vi "NEW数据采集传输系统.vi"() -> ()   [LabVIEW 2016, in "数据传输系统-06.lvlib"]
uses:
  <vilib>/Utility/miscctls.llb/LVPointTypeDef.ctl
  <vilib>/Utility/error.llb/whitespace.ctl
  <vilib>/picture/picture.llb/imagedata.ctl
  <vilib>/Utility/config.llb/NI_LVConfig.lvlib
  update/update.lvlib
panel:
  in  "共享MN":bool
  out "剖面数据补发":bool
  out "日志信息补发":bool
  out "数据补发":bool
  in  "自动更新":bool
  in  "数据补传":bool caption="确定"
  out "数据库打开失败次数":dbl
  out "与工控通信指示灯":bool
  in  "判断数据反馈":enum16{"非严格判断", "严格判断", "不判断"}(ring)
  in  "暂停上传":bool
  in  "配置表":bool caption="确定"
  in  "updateconfiguration":T1={"主机"="27.154.58.30", "用户"="update", "密码"="std23506", "远程路径"="数据传输系统\\平台数据传输系统.exe", "下载文件名"="平台数据传输系统.exe", "软件版本"=""}
  out "标题显示":string
  in  "更新":bool
  in  "系统编码选择框":string(combo)="地表水质量监测"
  in  "数据发送通道":enum16{"TCP", "VISA"}(ring)
  in  "baud rate":u32=9600 caption="波特率"
  in  "VISA resource name":refnum<visa-resource-name> caption="VISA资源名称"
  in  "实时数据发送时间间隔/min":i32=1
  in  "数据组合发送":bool
  in  "2011发送":bool
  in  "数据发送协议":enum16{"2005-212协议", "2017-212协议"}(ring)=enum."2017-212协议"
  in  "重发时间":T2(ring)
  in  "重发日期":T3(ring)
  in  "开机启动":bool
  in  "每周自动重发":bool=TRUE
  in  "确定":bool
  in  "返回":bool
  in  "PW":string
  in  "MN":string
  in  "PORT":string
  in  "IP":string
  in  "站点设备":string
  in  "站点名称":string
  out "设置超时时间/min":i32=1
  out "状态信息":T4={"1st Error to Convert "=63, "步骤 "=enum."发送数据", "元素"="实时数据", "TCP服务端掉线计数"=0, "TCP掉线时间节点"="2019/05/08 15:24:17"} {"1st Error to Convert" items=["无错误", "参数错误", "内存已满", "超出区域", "文件结束", "文件已打开", "一般文件IO错误", "未找到文件", "文件权限错误", "磁盘已满", "路径副本", "打开过多文件", "未启用", "未找到资源文件", "无法添加资源", "未找到资源", "未找到图像", "图像内存错误", "画笔不存在", "配置错误类型", "配置未找到解析段", "配置解析错误", "配置内存错误", "错误外部代码格式", "错误外部代码偏移量", "外部代码不存在", "空窗口", "销毁窗口错误", "空菜单", "打印已中止", "错误打印记录", "打印驱动程序错误", "打印时窗口错误", "打印时内存错误", "打印对话框错误", "一般打印错误", "无效设备引用句柄", "设备未找到", "设备参数错误", "设备单位错误", "无法打开设备", "设备调用已中止", "一般错误", "用户已取消", "对象ID过低", "对象ID过高", "对象不在堆中", "未知的堆", "错误DefProc ID", "DefProc不在表格中", "范围外信息", "空方法", "未知信息", "不支持管理器调用", "错误地址", "连接过程中", "连接超时", "连接过程中", "不支持网络属性", "网络错误", "正在使用的地址", "系统缺少内存", "连接已中止", "连接已拒绝", "连接未建立", "连接已建立", "连接已关闭", "初始化错误（交互应用程序管理器）", "错误事件发生", "等待无约束事件发生处理程序", "事件发生队列溢出", "错误路径", "未发出信号量", "未识别类型（交互应用程序管理器）"]}
  out "数据接收超时指示灯":bool
  out "空闲时间/s":string
  out "系统时间":string
  out "实时小时数据上传":bool
  out "系统状态改变":bool
  out "软件版本":string
  out "掉线指示":bool
  out "核查数据上传":bool
  out "配置信息":T5
  in  "参数配置":bool
  out "反控数据发送":bool
  out "读取报文显示":string
  out "发送报文显示":string
  out "心跳包":bool
  out "通信状态":bool
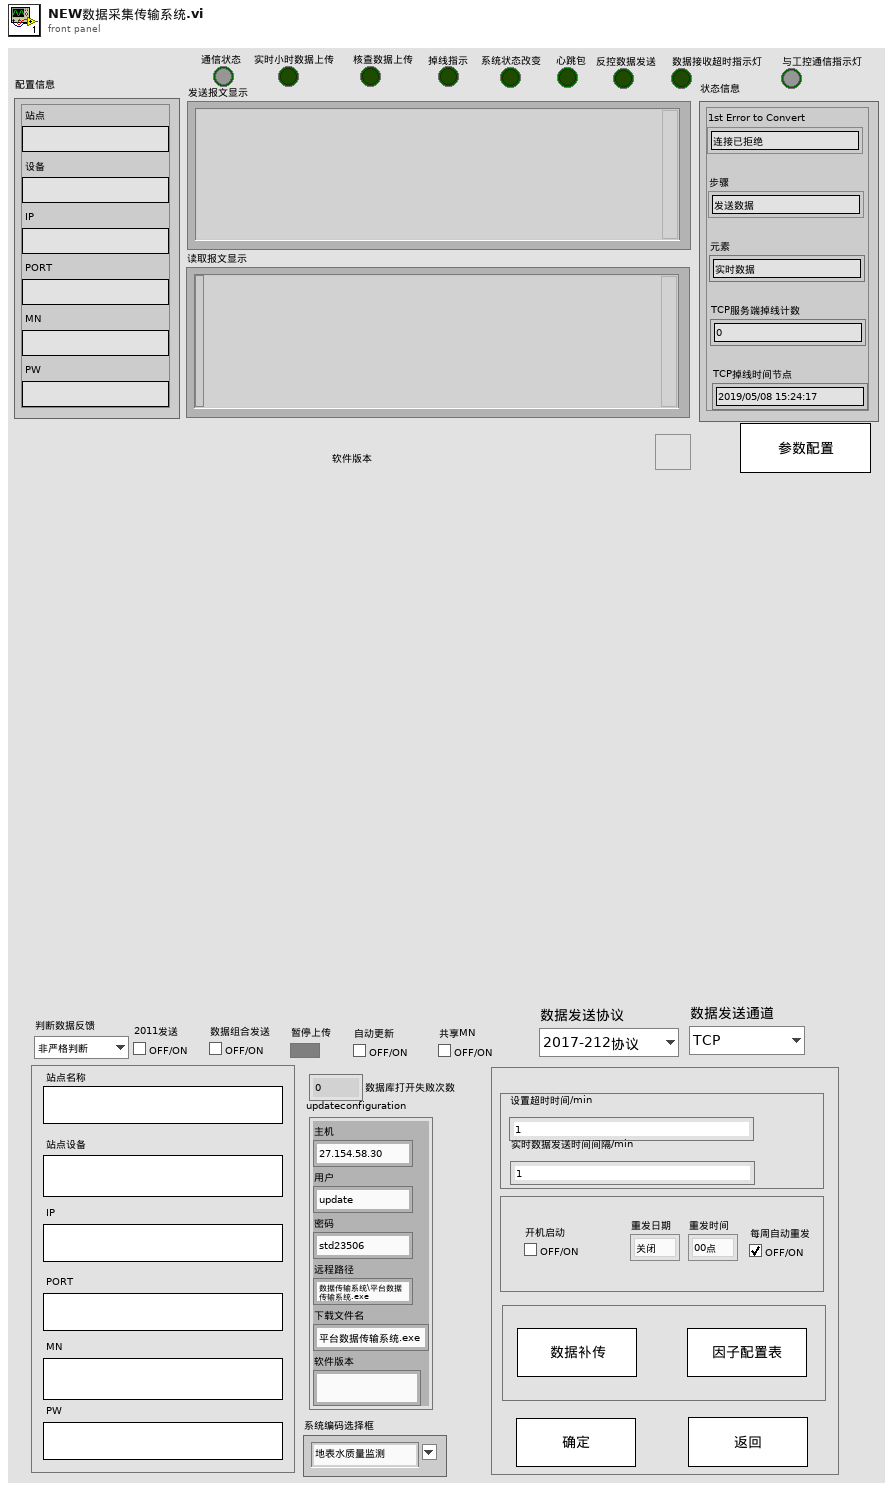
[diagram p1: front panel]
types:
  T1 = cluster{"主机":string, "用户":string, "密码":string, "远程路径":string, "下载文件名":string, "软件版本":string}
  T2 = enum16{"00点", "01点", "02点", "03点", "04点", "05点", "06点", "07点", "08点", "09点", "10点", "11点", "12点", "13点", "14点", "15点", "16点", "17点", "18点", "19点", "20点", "21点", "22点", "23点"}
  T3 = enum16{"关闭", "星期日", "星期一", "星期二", "星期三", "星期四", "星期五", "星期六"}
  T4 = cluster{"1st Error to Convert ":i32, "步骤 ":enum16{"打开连接", "发送数据", "读取数据", "数据处理", "关闭连接"}, "元素":string, "TCP服务端掉线计数":i32, "TCP掉线时间节点":string}
  T5 = cluster{"站点":string, "设备":string, "IP":string, "PORT":string, "MN":string, "PW":string}
  T6 = typedef "imagedata.ctl" = cluster{"image type":i32, "image depth":i32, "image":u8[], "mask":u8[], "colors":u32[], "Rectangle":cluster{"left":i16, "top":i16, "right":i16, "bottom":i16}}
  T7 = typedef "LVPointTypeDef.ctl" = cluster{"Horizontal":i16, "Vertical":i16}
  T8 = cluster{"setini":string, "sysini":string, "hechaini":string, "actualwrite":string, "actualread":string, "datasent":string, "反控命令信息队列":string, "反控与仪器交互":string}
  T9 = cluster{"配置表格[0]":string, "配置表格[1]":string, "配置表格[2]":string, "配置表格[3]":string, "配置表格[4]":string, "配置表格[5]":string, "配置表格[6]":string, "配置表格[7]":string, "配置表格[8]":string, "配置表格[9]":string, "配置表格[10]":string, "配置表格[11]":string, "配置表格[12]":string, "配置表格[13]":string, "配置表格[14]":string, "配置表格[15]":string, "配置表格[16]":string, "配置表格[17]":string, "配置表格[18]":string, "配置表格[19]":string, "配置表格[20]":string, "配置表格[21]":string, "配置表格[22]":string, "配置表格[23]":string, "配置表格[24]":string, "配置表格[25]":string, "配置表格[26]":string, "配置表格[27]":string, "配置表格[28]":string, "配置表格[29]":string, "配置表格[30]":string, "配置表格[31]":string, "配置表格[32]":string, "配置表格[33]":string, "配置表格[34]":string, "配置表格[35]":string, "配置表格[36]":string}
  T10 = cluster{"[0]":dbl, "[1]":dbl, "[2]":dbl, "[3]":dbl, "[4]":dbl, "[5]":dbl, "[6]":dbl, "[7]":dbl, "[8]":dbl, "[9]":dbl, "[10]":dbl, "[11]":dbl, "[12]":dbl, "[13]":dbl, "[14]":dbl, "[15]":dbl, "[16]":dbl, "[17]":dbl, "[18]":dbl, "[19]":dbl, "[20]":dbl, "[21]":dbl, "[22]":dbl, "[23]":dbl, "[24]":dbl, "[25]":dbl, "[26]":dbl, "[27]":dbl, "[28]":dbl, "[29]":dbl, "[30]":dbl, "[31]":dbl, "[32]":dbl, "[33]":dbl, "[34]":dbl, "[35]":dbl, "[36]":dbl}
  T11 = cluster{"时间标识":timestamp, "设备":string, "日志信息":string, "流程参数":string}
  T12 = typedef "NI_LVConfig.lvlib/Config Data RefNum.ctl" = refnum<k1>
  T13 = cluster{"CODMn":bool, "CODCr":bool, "DO":bool, "铜":bool, "PH":bool, "氨氮":bool, "比电导率":bool, "水温":bool, "COD":bool, "浊度":bool, "总氮":bool, "总磷":bool, "叶绿素a":bool, "藻密度":bool, "水位":bool, "流速":bool, "瞬时流量":bool, "累积流量":bool, "亚硝氮":bool, "硫化物":bool, "ORP":bool, "铅":bool, "镉":bool, "锌":bool, "镍":bool, "锰":bool, "汞":bool, "气温":bool, "气压":bool, "风速":bool, "风向":bool, "盐度":bool, "磷酸盐":bool, "硝氮":bool, "氟化物":bool, "挥发酚":bool, "氯化物":bool}
  T14 = cluster{"time1":string, "time2":string, "time3":string, "time4":string, "time5":string, "time6":string, "time7":string, "time8":string, "time9":string, "time10":string, "time11":string, "time12":string, "time13":string, "time14":string, "time15":string, "time16":string, "time17":string, "time18":string, "time19":string, "time20":string, "time21":string, "time22":string, "time23":string, "time24":string, "time25":string, "time26":string, "time27":string, "time28":string, "time29":string, "time30":string, "time31":string, "time32":string, "time33":string, "time34":string, "time35":string, "time36":string, "time37":string}
  T15 = cluster{"[0]":string, "[1]":string, "[2]":string, "[3]":string, "[4]":string, "[5]":string, "[6]":string, "[7]":string}
  T16 = cluster{"[0]":string, "[1]":string, "[2]":string, "[3]":string, "[4]":string, "[5]":string, "[6]":string, "[7]":string, "[8]":string, "[9]":string}
  T17 = cluster{"[0]":string, "[1]":string, "[2]":string, "[3]":string, "[4]":string, "[5]":string, "[6]":string}
  T18 = cluster{"[0]":string, "[1]":string, "[2]":string, "[3]":string, "[4]":string, "[5]":string, "[6]":string, "[7]":string, "[8]":string, "[9]":string, "[10]":string, "[11]":string, "[12]":string, "[13]":string, "[14]":string, "[15]":string, "[16]":string, "[17]":string}
  T19 = cluster{"[0]":string, "[1]":string, "[2]":string, "[3]":string, "[4]":string, "[5]":string, "[6]":string, "[7]":string, "[8]":string, "[9]":string, "[10]":string, "[11]":string, "[12]":string, "[13]":string, "[14]":string}
  T20 = cluster{"[0]":string, "[1]":string, "[2]":string, "[3]":string, "[4]":string, "[5]":string, "[6]":string, "[7]":string, "[8]":string, "[9]":string, "[10]":string, "[11]":string, "[12]":string, "[13]":string, "[14]":string, "[15]":string, "[16]":string, "[17]":string, "[18]":string, "[19]":string, "[20]":string, "[21]":string, "[22]":string, "[23]":string, "[24]":string, "[25]":string, "[26]":string, "[27]":string, "[28]":string, "[29]":string, "[30]":string, "[31]":string, "[32]":string, "[33]":string, "[34]":string, "[35]":string, "[36]":string}
  T21 = typedef "whitespace.ctl" = u16
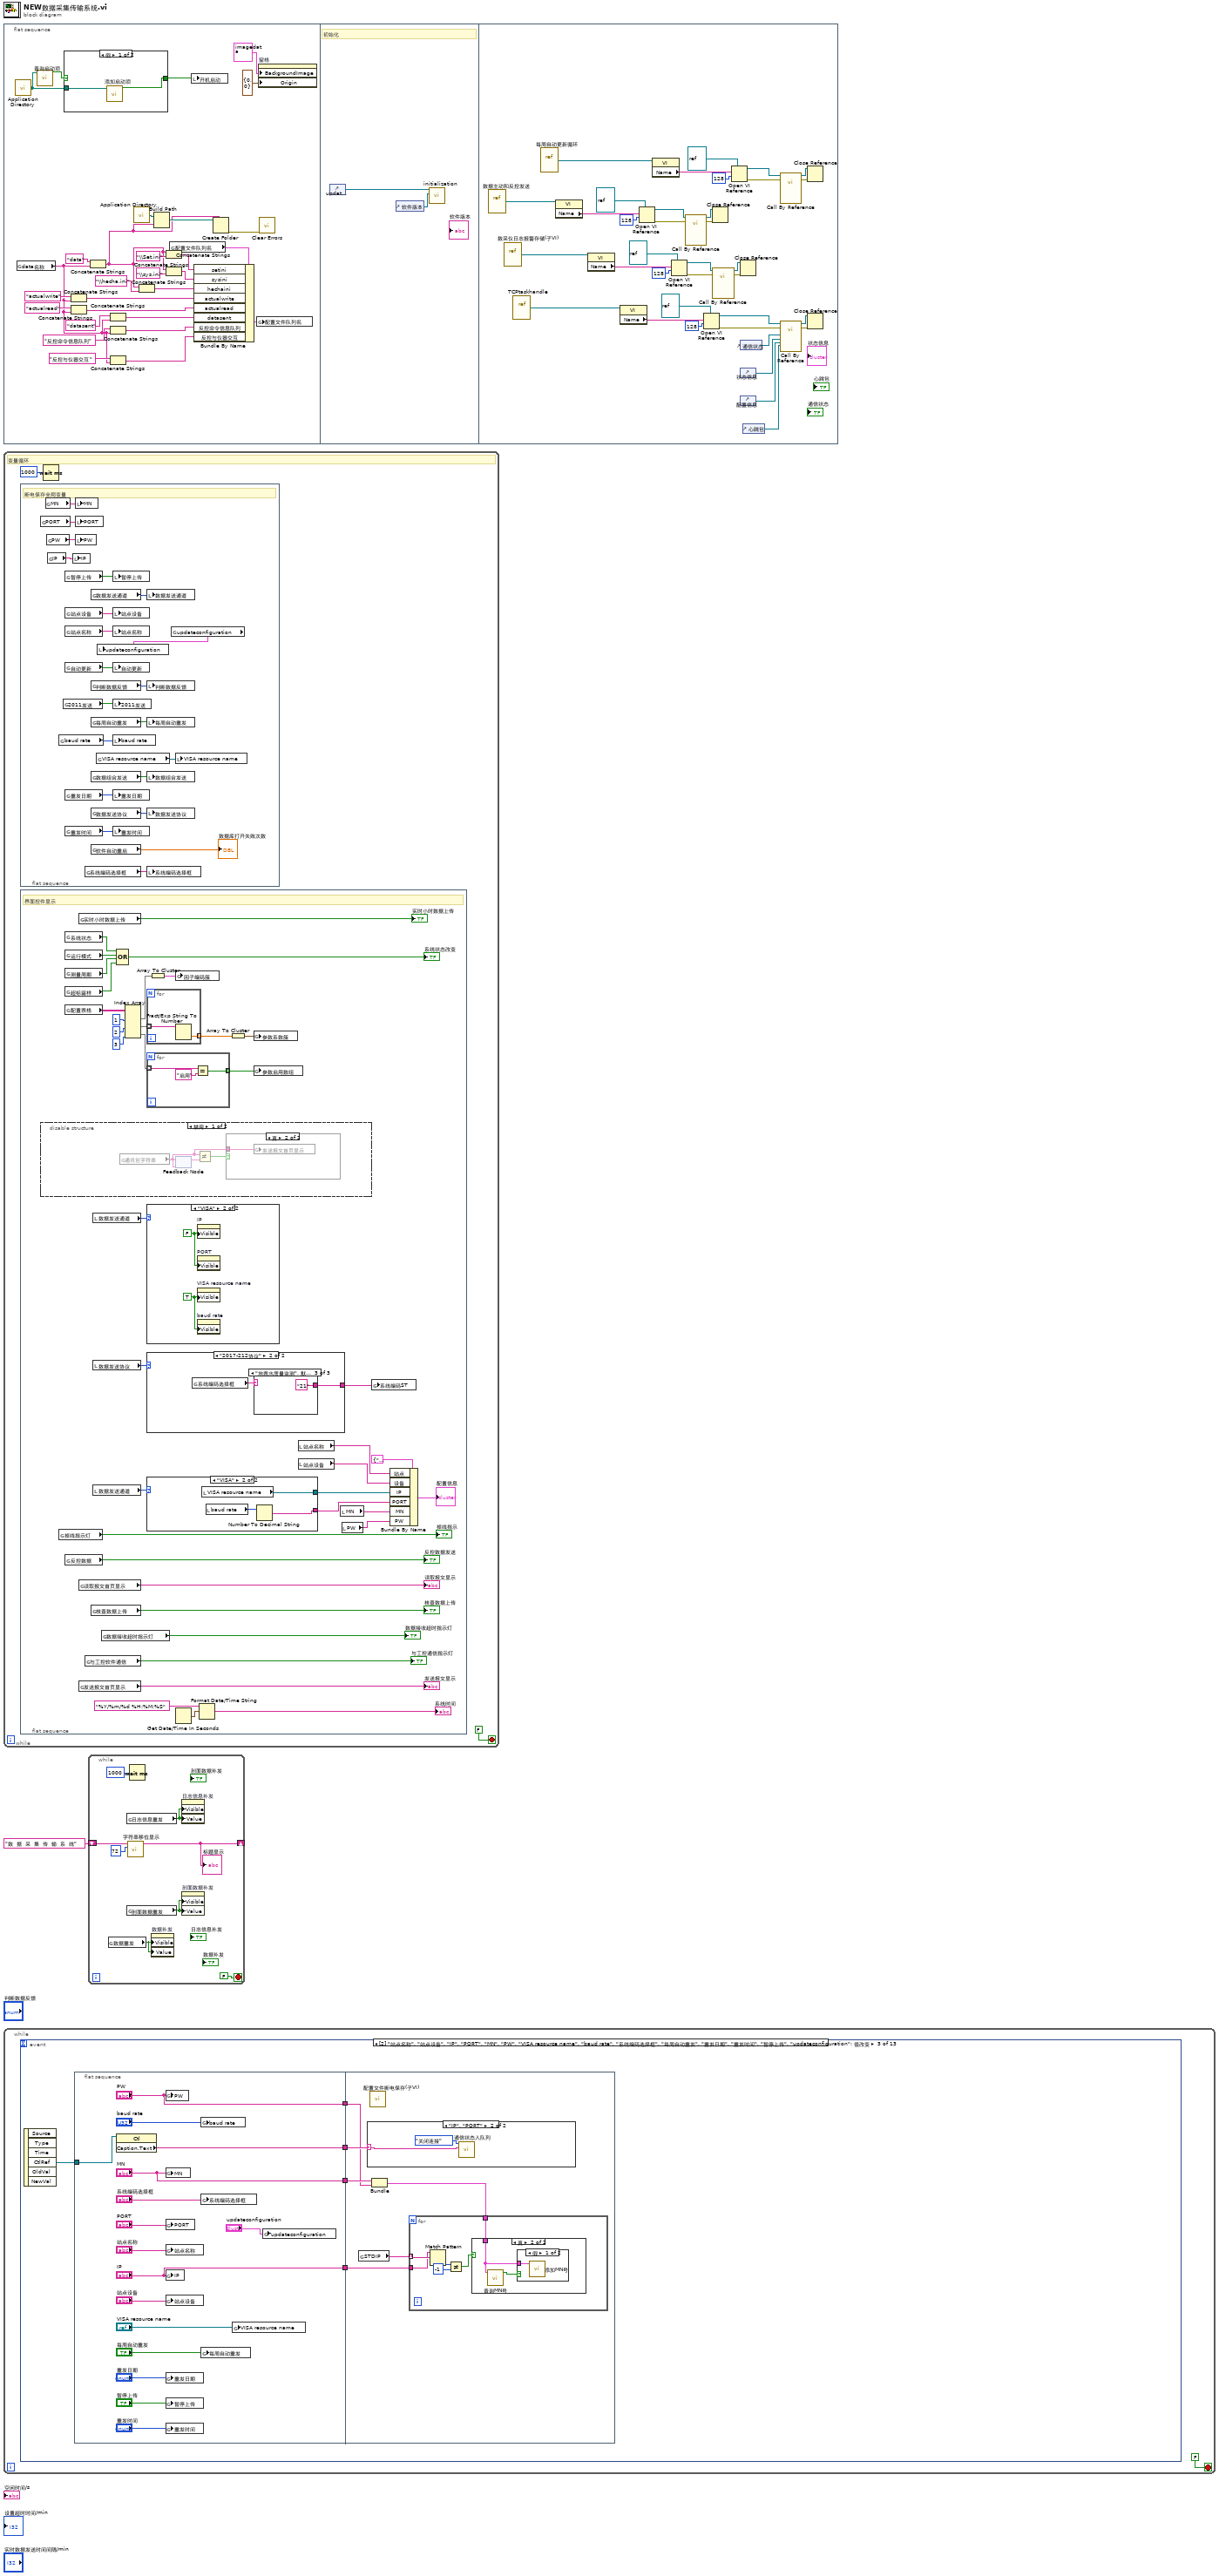
[diagram p0: block diagram]
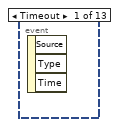
[diagram p2: hidden frame]
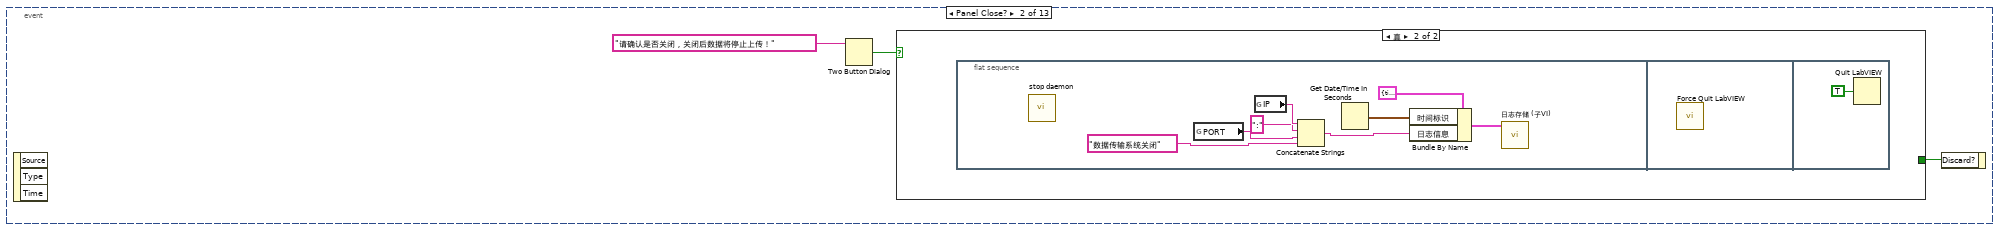
[diagram p3: hidden frame]
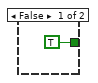
[diagram p4: hidden frame]
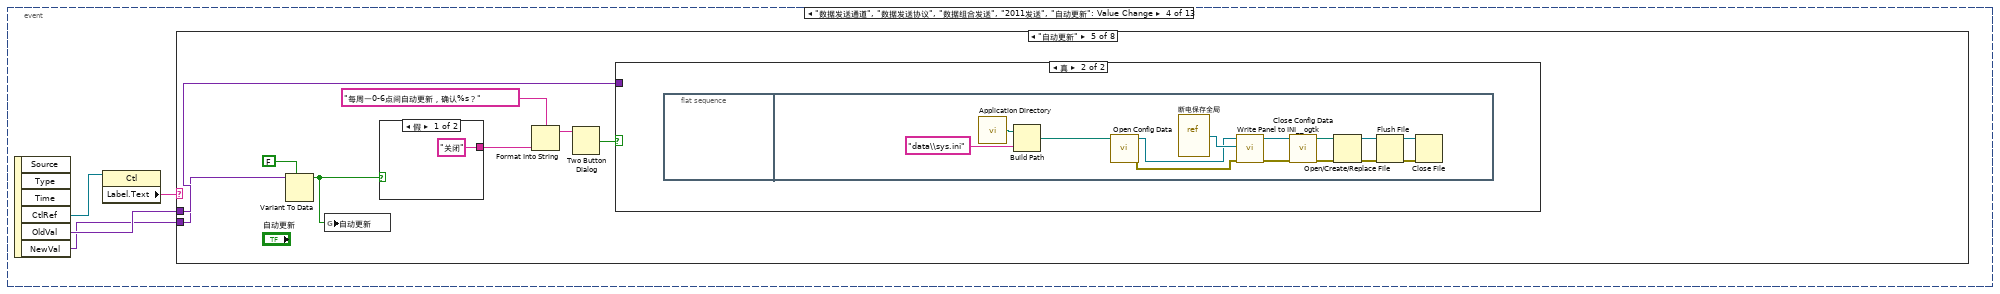
[diagram p8: hidden frame]
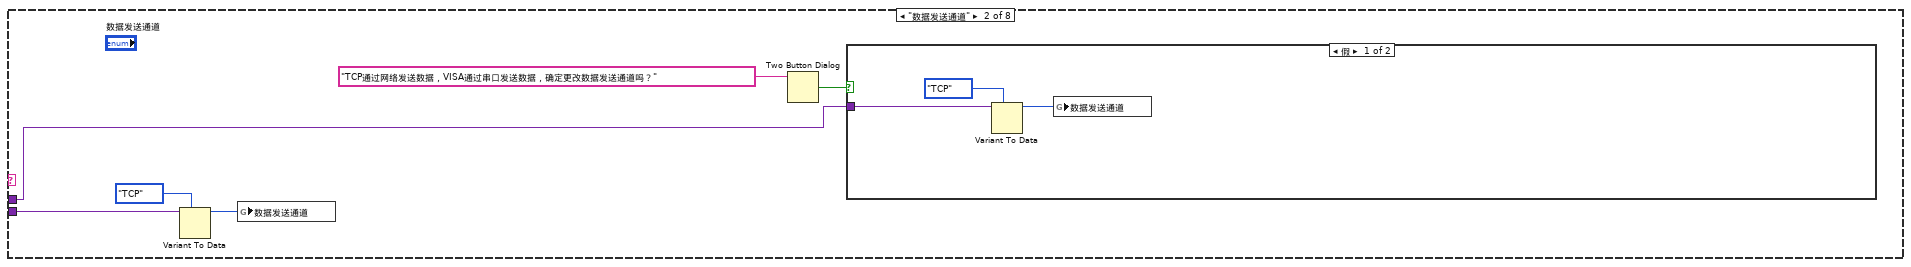
[diagram p10: hidden frame]
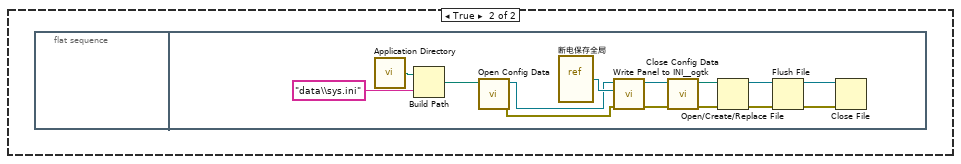
[diagram p11: hidden frame]
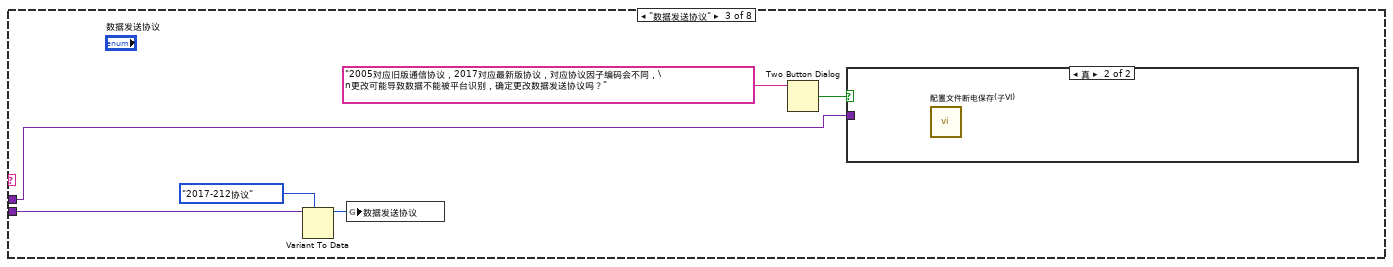
[diagram p12: hidden frame]
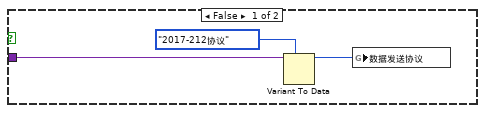
[diagram p13: hidden frame]
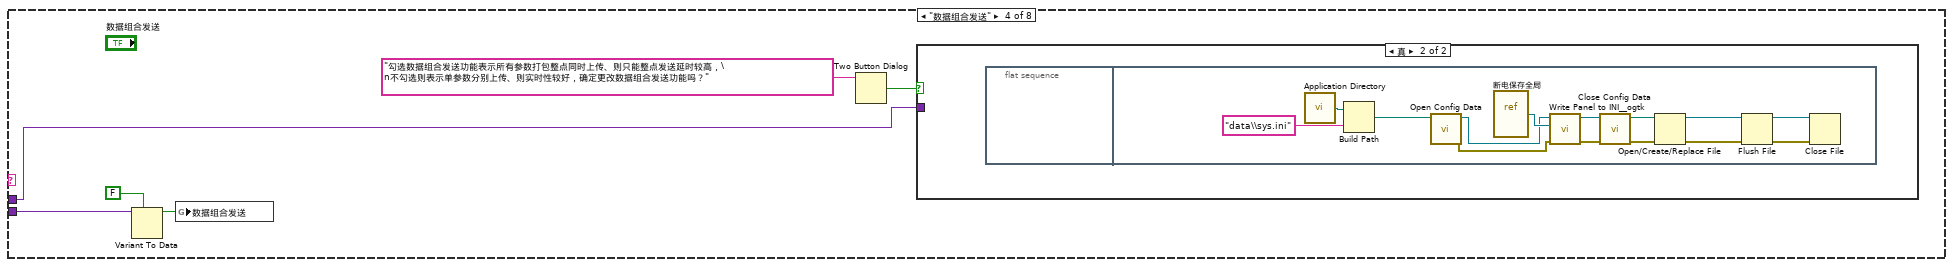
[diagram p14: hidden frame]
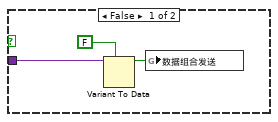
[diagram p15: hidden frame]
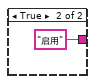
[diagram p16: hidden frame]
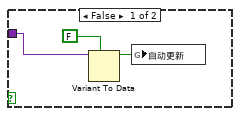
[diagram p17: hidden frame]
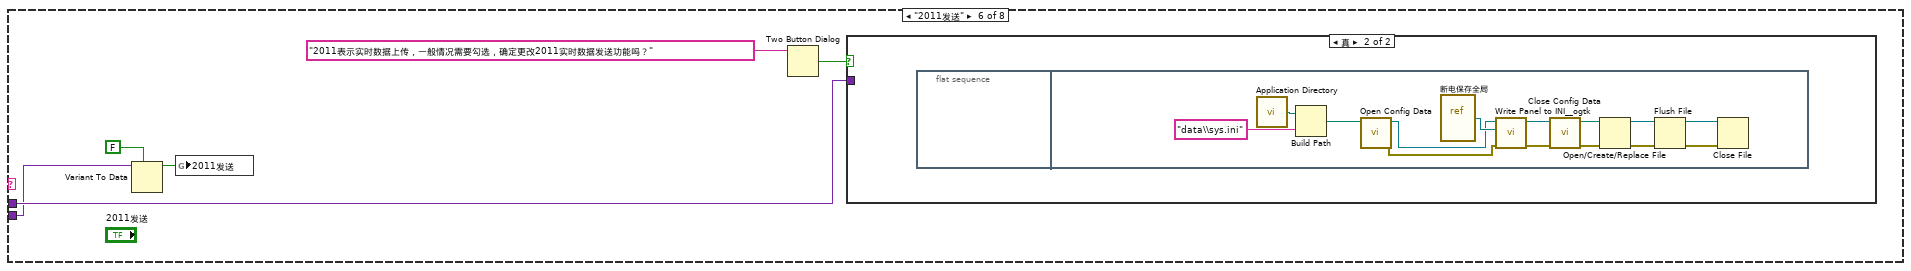
[diagram p18: hidden frame]
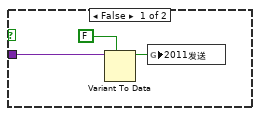
[diagram p19: hidden frame]
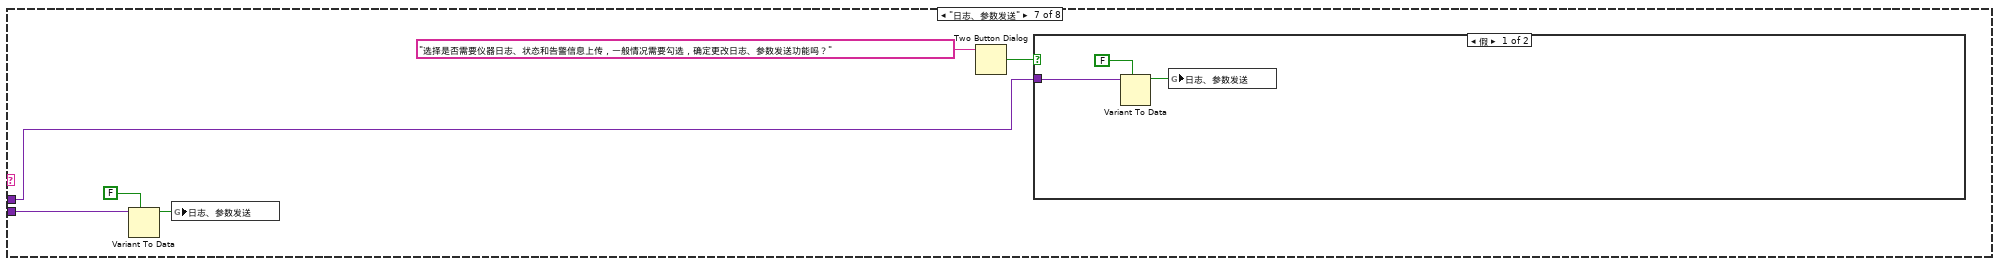
[diagram p20: hidden frame]
diagram:
  n1 = flat-sequence {
    frame #0 {
      n2 = call <vilib>:"Application Directory.vi"() -> ("Application Directory"=w8:path)
      n3 = global read "断电保存全局.vi" "data名称"() -> (w4:string)
      n4 = call "查询启动项.vi"("启动文件路径"=w8) -> ("包含启动项"=w7:bool)  [unwired: 9 in, 1 out]
      n5 = case shown="假" w7 {
        selector: w7 -> [_ w33]
        tunnel: w8 -> [w32 _]
        tunnel: [w31 w33] -> w6
        frame False {
          n6 = call "添加启动项.vi"("启动文件路径"=w32) -> ("添加成功标记"=w31:bool)  [unwired: 9 in, 1 out]
        }
        frame True {
        }
      }
      n7 = Concatenate Strings("actualwrite" ("名称（未命名）"), w4) -> (w18:string)
      n8 = Concatenate Strings("actualread" ("名称（未命名）"), w4) -> (w16:string)
      n9 = Concatenate Strings("data" ("对话框窗口（创建文件夹）"), w4) -> (w23:string)
      n10 = Concatenate Strings("datasent" ("名称（未命名）"), w4) -> (w14:string)
      n11 = Concatenate Strings("反控命令信息队列" ("名称（未命名）"), w4) -> (w10:string)
      n12 = Concatenate Strings("反控与仪器交互" ("名称（未命名）"), w4) -> (w11:string)
      n13 = call <vilib>:"Application Directory.vi"() -> ("Application Directory"=w29:path)
      n14 = Concatenate Strings(w23, "\\hecha.ini" ("名称或相对路径")) -> (w21:string)
      n15 = Build Path(base path=w29, name or relative path=w23) -> (appended path=w28:path)
      n16 = Concatenate Strings(w23, "\\Set.ini" ("名称或相对路径")) -> (w25:string)
      n17 = Concatenate Strings(w23, "\\sys.ini" ("名称或相对路径")) -> (w22:string)
      n18 = global read "全局1.vi" "配置文件队列名"() -> (w2:T8)
      n19 = local write "开机启动"(w6) -> ()
      n20 = Bundle By Name(cluster=w2, "setini"=w25, "sysini"=w22, "hechaini"=w21, "actualwrite"=w18, "actualread"=w16, "datasent"=w14, "反控命令信息队列"=w10, "反控与仪器交互"=w11) -> (w3:T8)
      n21 = Create Folder(prompt (Create Folder)=w23, path (use dialog)=w28) -> (error out=w27:errorcluster)  [unwired: 1 in, 2 out]
      n22 = global write "全局1.vi" "配置文件队列名"(w3) -> ()
      n23 = property on="窗格" class="Pane"("BackgroundImage"=T6 {"image type"=0, "image depth"=24, "image"=array[12288000 elements], "mask"=[], "colors"=[], "Rectangle"={"left"=0, "top"=0, "right"=2560, "bottom"=1600}} ("image data"), "Origin"=T7 {"Horizontal"=0, "Vertical"=0} ("原点")) -> ()  [unwired: 2 in, 2 out]
      n24 = call <vilib>:"Clear Errors.vi"("error in (no error)"=w27) -> ()  [unwired: 5 in, 2 out]
    }
    frame #1 {
      # "初始化"
      n25 = control-ref of="updateconfiguration"() -> (w35:refnum<vi>)
      n26 = control-ref of="软件版本"() -> (w34:refnum<vi>)
      n27 = call "initialization.vi"("软件版本"=w34, "updateconfiguration"=w35) -> ()  [unwired: 9 in]
    }
    frame #2 {
      n28 = vi-ref "数据主动和反控发送.vi"() -> (w63:refnum<vi>)
      n29 = vi-ref "数采仪日志报警存储(子VI).vi"() -> (w64:refnum<vi>)
      n30 = vi-ref "TCPtaskhandle.vi"() -> (w40:refnum<vi>)
      n31 = vi-ref "每周自动更新循环.vi"() -> (w55:refnum<vi>)
      n32 = property class="VI"(reference=w63) -> ("Name"=w62:string)  [unwired: 1 in, 2 out]
      n33 = property class="VI"(reference=w64) -> ("Name"=w71:string)  [unwired: 1 in, 2 out]
      n34 = property class="VI"(reference=w40) -> ("Name"=w47:string)  [unwired: 1 in, 2 out]
      n35 = Open VI Reference(type specifier VI Refnum (for type only)=refnum<vi> refnum, vi path=w62, options=128 ("选项")) -> (vi reference=w60:refnum<vi>, error out=w58:errorcluster)  [unwired: 3 in]
      n36 = property class="VI"(reference=w55) -> ("Name"=w48:string)  [unwired: 1 in, 2 out]
      n37 = Open VI Reference(type specifier VI Refnum (for type only)=refnum<vi> refnum, vi path=w71, options=128 ("选项")) -> (vi reference=w69:refnum<vi>, error out=w67:errorcluster)  [unwired: 3 in]
      n38 = call-by-ref "?"(reference=w60, error in=w58) -> (reference out=w56:refnum<vi>, error out=w57:errorcluster)  [unwired: 12 in]
      n39 = Open VI Reference(type specifier VI Refnum (for type only)=refnum<vi> refnum, vi path=w47, options=128 ("选项")) -> (vi reference=w45:refnum<vi>, error out=w43:errorcluster)  [unwired: 3 in]
      n40 = Close Reference(reference=w56, error in (no error)=w57) -> ()  [unwired: 1 out]
      n41 = call-by-ref "?"(reference=w69, error in=w67) -> (reference out=w65:refnum<vi>, error out=w66:errorcluster)  [unwired: 12 in]
      n42 = Open VI Reference(type specifier VI Refnum (for type only)=refnum<vi> refnum, vi path=w48, options=128 ("选项")) -> (vi reference=w50:refnum<vi>, error out=w52:errorcluster)  [unwired: 3 in]
      n43 = Close Reference(reference=w65, error in (no error)=w66) -> ()  [unwired: 1 out]
      n44 = control-ref of="通信状态"() -> (w39:refnum<vi>)
      n45 = control-ref of="状态信息"() -> (w38:refnum<vi>)
      n46 = control-ref of="配置信息"() -> (w37:refnum<vi>)
      n47 = control-ref of="心跳包"() -> (w36:refnum<vi>)
      n48 = call-by-ref "?"(reference=w50, error in=w52) -> (reference out=w54:refnum<vi>, error out=w53:errorcluster)  [unwired: 12 in]
      n49 = call-by-ref "?"(reference=w45, error in=w43, "心跳包"=w36, "配置信息"=w37, "状态信息"=w38, "通信状态"=w39) -> (reference out=w41:refnum<vi>, error out=w42:errorcluster)  [unwired: 8 in]
      n50 = Close Reference(reference=w54, error in (no error)=w53) -> ()  [unwired: 1 out]
      n51 = Close Reference(reference=w41, error in (no error)=w42) -> ()  [unwired: 1 out]
    }
  }
  n52 = while {
    stop <- FALSE stop-if-true
    # "变量循环"
    n53 = flat-sequence {
      frame #0 {
        # "断电保存全局变量"
        n54 = global read "断电保存全局.vi" "PORT"() -> (w158:string)
        n55 = global read "断电保存全局.vi" "MN"() -> (w157:string)
        n56 = global read "断电保存全局.vi" "PW"() -> (w156:string)
        n57 = global read "断电保存全局.vi" "IP"() -> (w159:string)
        n58 = global read "断电保存全局.vi" "baud rate"() -> (w154:u32)
        n59 = global read "断电保存全局.vi" "2011发送"() -> (w150:bool)
        n60 = global read "断电保存全局.vi" "暂停上传"() -> (w144:bool)
        n61 = global read "断电保存全局.vi" "站点设备"() -> (w160:string)
        n62 = global read "断电保存全局.vi" "站点名称"() -> (w161:string)
        n63 = global read "断电保存全局.vi" "自动更新"() -> (w142:bool)
        n64 = global read "断电保存全局.vi" "重发日期"() -> (w152:T3)
        n65 = global read "断电保存全局.vi" "重发时间"() -> (w145:T2)
        n66 = local write "IP"(w159) -> ()
        n67 = local write "MN"(w157) -> ()
        n68 = local write "PORT"(w158) -> ()
        n69 = local write "PW"(w156) -> ()
        n70 = global read "断电保存全局.vi" "系统编码选择框"() -> (w146:string)
        n71 = global read "断电保存全局.vi" "数据发送通道"() -> (w147:enum16{"TCP", "VISA"})
        n72 = global read "断电保存全局.vi" "判断数据反馈"() -> (w151:enum16{"非严格判断", "严格判断", "不判断"})
        n73 = global read "断电保存全局.vi" "每周自动重发"() -> (w153:bool)
        n74 = global read "断电保存全局.vi" "数据组合发送"() -> (w149:bool)
        n75 = global read "断电保存全局.vi" "数据发送协议"() -> (w148:enum16{"2005-212协议", "2017-212协议"})
        n76 = global read "全局1.vi" "软件自动重启"() -> (→"数据库打开失败次数":dbl)
        n77 = global read "断电保存全局.vi" "VISA resource name"() -> (w155:refnum<visa-resource-name>)
        n78 = local write "暂停上传"(w144) -> ()
        n79 = local write "站点设备"(w160) -> ()
        n80 = local write "站点名称"(w161) -> ()
        n81 = local write "自动更新"(w142) -> ()
        n82 = local write "2011发送"(w150) -> ()
        n83 = local write "baud rate"(w154) -> ()
        n84 = local write "重发日期"(w152) -> ()
        n85 = local write "重发时间"(w145) -> ()
        n86 = local write "数据发送通道"(w147) -> ()
        n87 = local write "判断数据反馈"(w151) -> ()
        n88 = local write "每周自动重发"(w153) -> ()
        n89 = local write "数据组合发送"(w149) -> ()
        n90 = local write "数据发送协议"(w148) -> ()
        n91 = local write "系统编码选择框"(w146) -> ()
        n92 = global read "断电保存全局.vi" "updateconfiguration"() -> (w141:T1)
        n93 = local write "updateconfiguration"(w141) -> ()
        n94 = local write "VISA resource name"(w155) -> ()
      }
    }
    n95 = flat-sequence {
      frame #0 {
        # "界面控件显示"
        n96 = disable-structure shown="禁用" {
          frame Disabled {
            n97 = global read "全局1.vi" "通讯包字符串"() -> (w114:string)
            n98 = feedback #1(w114) -> (w115:string)
            n99 = feedback-in #1(w114) -> ()
            n100 = Not Equal?(x=w114, y=w115) -> (x != y?=w113:bool)
            n101 = case shown="真" w113 {
              tunnel: w114 -> [_ w116]
              frame False {
              }
              frame True {
                n102 = global write "全局1.vi" "发送报文首页显示"(w116) -> ()
              }
            }
          }
          frame Enabled {
          }
        }
        n103 = global read "全局 数据发送重叠.vi" "掉线指示灯"() -> (→"掉线指示":bool)
        n104 = global read "全局1.vi" "系统状态"() -> (w86:bool)
        n105 = global read "全局1.vi" "运行模式"() -> (w87:bool)
        n106 = global read "全局1.vi" "测量周期"() -> (w88:bool)
        n107 = global read "全局1.vi" "超标留样"() -> (w89:bool)
        n108 = global read "断电保存全局.vi" "配置表格"() -> (w84:string[][])
        n109 = global read "全局1.vi" "反控数据"() -> (→"反控数据发送":bool)
        n110 = global read "全局1.vi" "实时小时数据上传"() -> (→"实时小时数据上传":bool)
        n111 = global read "全局1.vi" "读取报文首页显示"() -> (→"读取报文显示":string)
        n112 = global read "全局1.vi" "发送报文首页显示"() -> (→"发送报文显示":string)
        n113 = global read "全局1.vi" "与工控软件通信"() -> (→"与工控通信指示灯":bool)
        n114 = global read "全局1.vi" "核查数据上传"() -> (→"核查数据上传":bool)
        n115 = local read "数据发送通道"() -> (w94:enum16{"TCP", "VISA"})
        n116 = local read "数据发送协议"() -> (w101:enum16{"2005-212协议", "2017-212协议"})
        n117 = local read "数据发送通道"() -> (w112:enum16{"TCP", "VISA"})
        n118 = global read "全局 数据发送重叠.vi" "数据接收超时指示灯"() -> (→"数据接收超时指示灯":bool)
        n119 = Compound Arithmetic op=OR ("复合运算")(w86, w87, w88, w89) -> (→"系统状态改变":bool)
        n120 = Index Array(array=w84, index (col) #1=1 ("禁用的索引 (列)"), index (col) #2=2 ("索引 (列)"), index (col) #3=3 ("索引 (列)")) -> (element #1=w82:string[], element #2=w76:string[], element #3=w78:string[])  [unwired: 3 in]
        n121 = for {
          tunnel: w76 -> [w118] mode=indexing
          tunnel: [w117] -> w75 mode=indexing
          n122 = Fract/Exp String To Number(string=w118) -> (number=w117:dbl)  [unwired: 3 in, 1 out]
        }
        n123 = for {
          tunnel: w78 -> [w121] mode=indexing
          tunnel: [w119] -> w77 mode=indexing
          n124 = Equal?(x=w121, y="启用") -> (x = y?=w119:bool)
        }
        n125 = case shown="\"VISA\"" w94 {
          frame "TCP", Default {
            w122 = TRUE ("可见")
            w123 = FALSE ("可见")
            n126 = property on="IP" class="Str"("Visible"=w122) -> ()  [unwired: 2 in, 2 out]
            n127 = property on="PORT" class="Str"("Visible"=w122) -> ()  [unwired: 2 in, 2 out]
            n128 = property on="VISA resource name" class="VISAName"("Visible"=w123) -> ()  [unwired: 2 in, 2 out]
            n129 = property on="baud rate" class="DigNum (严格)"("Visible"=w123) -> ()  [unwired: 2 in, 2 out]
          }
          frame "VISA" {
            w124 = FALSE ("可见")
            w125 = TRUE ("可见")
            n130 = property on="IP" class="Str"("Visible"=w124) -> ()  [unwired: 2 in, 2 out]
            n131 = property on="PORT" class="Str"("Visible"=w124) -> ()  [unwired: 2 in, 2 out]
            n132 = property on="VISA resource name" class="VISAName"("Visible"=w125) -> ()  [unwired: 2 in, 2 out]
            n133 = property on="baud rate" class="DigNum (严格)"("Visible"=w125) -> ()  [unwired: 2 in, 2 out]
          }
        }
        n134 = case shown="\"2017-212协议\"" w101 {
          tunnel: [w126 w131] -> w100
          frame "2005-212协议", Default {
            n135 = global read "断电保存全局.vi" "系统编码选择框"() -> (w127:string)
            n136 = case shown="\"地表水体污染源\"" w127 {
              tunnel: ["52" ("设备编码MN") "32" ("设备编码MN") "21" ("设备编码MN")] -> w126
              frame "污水排放过程监测" {
              }
              frame "地表水体污染源" {
              }
              frame "地表水质量监测", Default {
              }
            }
          }
          frame "2017-212协议" {
            n137 = global read "断电保存全局.vi" "系统编码选择框"() -> (w132:string)
            n138 = case shown="\"地表水质量监测\", 默认" w132 {
              tunnel: ["52" ("设备编码MN") "32" ("设备编码MN") "21" ("设备编码MN")] -> w131
              frame "污水排放过程监测" {
              }
              frame "地表水体污染源" {
              }
              frame "地表水质量监测", Default {
              }
            }
          }
        }
        n139 = case shown="\"VISA\"" w112 {
          tunnel: [w137 w140] -> w109
          tunnel: [w136 w138] -> w106
          frame "TCP", Default {
            n140 = local read "PORT"() -> (w136:string)
            n141 = local read "IP"() -> (w137:string)
          }
          frame "VISA" {
            n142 = local read "VISA resource name"() -> (w140:refnum<visa-resource-name>)
            n143 = local read "baud rate"() -> (w139:u32)
            n144 = Number To Decimal String(number=w139) -> (decimal integer string=w138:string)  [unwired: 1 in]
          }
        }
        n145 = Array To Cluster(array=w82) -> (cluster=w85:T9)
        n146 = global write "断电保存全局.vi" "因子编码簇"(w85) -> ()
        n147 = Get Date/Time In Seconds() -> (seconds since 1Jan1904=w102:timestamp)
        n148 = Format Date/Time String(time format string (%c)="%Y/%m/%d %H:%M:%S" ("时间格式字符串(%c)"), seconds (now)=w102) -> (date/time string=→"系统时间":string)  [unwired: 1 in]
        n149 = Array To Cluster(array=w75) -> (cluster=w79:T10)
        n150 = global write "断电保存全局.vi" "参数系数簇"(w79) -> ()
        n151 = global write "断电保存全局.vi" "参数启用数组"(w77) -> ()
        n152 = local read "站点名称"() -> (w108:string)
        n153 = local read "站点设备"() -> (w107:string)
        n154 = local read "MN"() -> (w105:string)
        n155 = local read "PW"() -> (w104:string)
        n156 = global write "全局1.vi" "系统编码ST"(w100) -> ()
        n157 = Bundle By Name(cluster=T5 {"站点"="", "设备"="", "IP"="", "PORT"="", "MN"="", "PW"=""} ("配置信息"), "站点"=w108, "设备"=w107, "IP"=w109, "PORT"=w106, "MN"=w105, "PW"=w104) -> (→"配置信息":T5)
      }
    }
    n158 = Wait (ms)(milliseconds to wait=u32 1000 ("等待时间（毫秒）")) -> ()  [unwired: 1 out]
  }
  n159 = while {
    stop <- FALSE stop-if-true
    n160 = event shown="[2] \"站点名称\", \"站点设备\", \"IP\", \"PORT\", \"MN\", \"PW\", \"VISA resource name\", \"baud rate\", \"系统编码选择框\", \"每周自动重发\", \"重发日期\", \"重发时间\", \"暂停上传\", \"updateconfiguration\": 值改变" {
      selector: _ -> [_ _ _ _ _ _ _ _ _ _ _ _ _]
      dyn-events: _ -> [_ _ _ _ _ _ _ _ _ _ _ _ _]
      timeout: _ -> [_ _ _ _ _ _ _ _ _ _ _ _ _]
      event Timeout {
        n161 = event-data() -> ()  [unwired: 1 in, 3 out]
      }
      event Panel Close? {
        n162 = event-data() -> ()  [unwired: 1 in, 3 out]
        n163 = Two Button Dialog(message="请确认是否关闭，关闭后数据将停止上传！" ("消息")) -> (T button?=w164:bool)  [unwired: 2 in]
        n164 = case shown="真" w164 {
          tunnel: [TRUE _] -> w163
          frame False {
          }
          frame True {
            n165 = flat-sequence {
              frame #0 {
                n166 = call "stop daemon.vi"() -> ()  [unwired: 11 in, 1 out]
                n167 = global read "断电保存全局.vi" "PORT"() -> (w170:string)
                n168 = global read "断电保存全局.vi" "IP"() -> (w172:string)
                n169 = Concatenate Strings(w172, ":", w170, "数据传输系统关闭" ("日志信息")) -> (w168:string)
                n170 = Get Date/Time In Seconds() -> (seconds since 1Jan1904=w174:timestamp)
                n171 = Bundle By Name(cluster=T11 {"时间标识"=timestamp(0 s since 1904-01-01), "设备"="数采仪", "日志信息"="", "流程参数"=""} ("data in"), "时间标识"=w174, "日志信息"=w168) -> (w173:T11)
                n172 = call "日志存储 (子VI).vi"("data in"=w173) -> ()  [unwired: 11 in]
              }
              frame #1 {
                n173 = call "Force Quit LabVIEW.vi"() -> ()  [unwired: 10 in, 2 out]
              }
              frame #2 {
                n174 = Quit LabVIEW(quit? (T)=TRUE ("退出？(T)")) -> ()
              }
            }
          }
        }
        n175 = event-data("Discard?"=w163) -> ()  [unwired: 1 in, 1 out]
      }
      event "站点名称", "站点设备", "IP", "PORT", "MN", "PW", "VISA resource name", "baud rate", "系统编码选择框", "每周自动重发", "重发日期", "重发时间", "暂停上传", "updateconfiguration": Value Change {
        n176 = event-data() -> ("CtlRef"=w180:refnum<vi>)  [unwired: 1 in, 5 out]
        n177 = flat-sequence {
          tunnel: w180 -> [w186]
          tunnel: [w185] -> w179
          tunnel: ["IP"] -> w178
          tunnel: ["MN"] -> w177
          tunnel: ["PW"] -> w176
          tunnel: w179 -> [w202]
          tunnel: w178 -> [w200]
          tunnel: w177 -> [w199]
          tunnel: w176 -> [w198]
          frame #0 {
            n178 = property class="Ctl"(reference=w186) -> ("Caption.Text"=w185:string)  [unwired: 1 in, 2 out]
            n179 = global write "断电保存全局.vi" "PW"("PW") -> ()
            n180 = global write "断电保存全局.vi" "MN"("MN") -> ()
            n181 = global write "断电保存全局.vi" "PORT"("PORT") -> ()
            n182 = global write "断电保存全局.vi" "站点名称"("站点名称") -> ()
            n183 = global write "断电保存全局.vi" "IP"("IP") -> ()
            n184 = global write "断电保存全局.vi" "站点设备"("站点设备") -> ()
            n185 = global write "断电保存全局.vi" "重发日期"("重发日期") -> ()
            n186 = global write "断电保存全局.vi" "暂停上传"("暂停上传") -> ()
            n187 = global write "断电保存全局.vi" "重发时间"("重发时间") -> ()
            n188 = global write "断电保存全局.vi" "baud rate"("baud rate") -> ()
            n189 = global write "断电保存全局.vi" "系统编码选择框"("系统编码选择框") -> ()
            n190 = global write "断电保存全局.vi" "每周自动重发"("每周自动重发") -> ()
            n191 = global write "断电保存全局.vi" "VISA resource name"("VISA resource name") -> ()
            n192 = global write "断电保存全局.vi" "updateconfiguration"("updateconfiguration") -> ()
          }
          frame #1 {
            n193 = global read "断电保存全局.vi" "STDIP"() -> (w201:string[])
            n194 = case shown="\"IP\", \"PORT\"" w202 {
              selector: w202 -> [_ w212]
              frame "假", Default {
              }
              frame "IP", "PORT" {
                n195 = call "通信状态入队列.vi"("发送报文"=w212, "枚举"=enum16{"打开连接", "发送数据", "读取数据", "数据处理", "关闭连接"}."关闭连接") -> ()  [unwired: 9 in, 1 out]
              }
            }
            n196 = call "配置文件断电保存(子VI).vi"() -> ()  [unwired: 12 in]
            n197 = Bundle("MN"=w199, "PW"=w198) -> (w197:cluster{"MN":string, "PW":string})  [unwired: 1 in]
            n198 = for {
              tunnel: w201 -> [w208] mode=indexing
              tunnel: w200 -> [w207]
              tunnel: w197 -> [w203]
              n199 = Match Pattern(string=w207, regular expression=w208) -> (offset past match=w206:i32)  [unwired: 1 in, 3 out]
              n200 = Not Equal?(x=w206, y=-1) -> (x != y?=w204:bool)
              n201 = case shown="真" w204 {
                tunnel: w203 -> [_ w210]
                frame False {
                }
                frame True {
                  n202 = call "查询MN号.vi"("簇"=w210) -> ("包含启动项"=w209:bool)  [unwired: 9 in, 1 out]
                  n203 = case shown="假" w209 {
                    tunnel: w210 -> [w211 _]
                    frame False {
                      n204 = call "添加MN号.vi"("簇"=w211) -> ()  [unwired: 9 in, 2 out]
                    }
                    frame True {
                    }
                  }
                }
              }
            }
          }
        }
      }
      event "数据发送通道", "数据发送协议", "数据组合发送", "2011发送", "自动更新": Value Change {
        n205 = event-data() -> ("CtlRef"=w217:refnum<vi>, "OldVal"=w215:variant, "NewVal"=w214:variant)  [unwired: 1 in, 3 out]
        n206 = property class="Ctl"(reference=w217) -> ("Label.Text"=w216:string)  [unwired: 1 in, 2 out]
        n207 = case shown="\"自动更新\"" w216 {
          tunnel: w215 -> [_ w221 w244 w253 w279 w303 w326 w347]
          tunnel: w214 -> [_ w218 w241 w250 w277 w300 w323 w346]
          frame "假", Default {
          }
          frame "数据发送通道" {
            n208 = Variant To Data(type=enum16{"TCP", "VISA"}."TCP" ("数据发送通道"), Variant=w218) -> (data=w219:enum16{"TCP", "VISA"})  [unwired: 1 in, 1 out]
            n209 = global write "断电保存全局.vi" "数据发送通道"(w219) -> ()
            n210 = Two Button Dialog(message="TCP通过网络发送数据，VISA通过串口发送数据，确定更改数据发送通道吗？" ("消息")) -> (T button?=w222:bool)  [unwired: 2 in]
            n211 = case shown="假" w222 {
              tunnel: w221 -> [w225 _]
              frame False {
                n212 = Variant To Data(type=enum16{"TCP", "VISA"}."TCP" ("数据发送通道"), Variant=w225) -> (data=w224:enum16{"TCP", "VISA"})  [unwired: 1 in, 1 out]
                n213 = global write "断电保存全局.vi" "数据发送通道"(w224) -> ()
              }
              frame True {
                n214 = flat-sequence {
                  frame #0 {
                  }
                  frame #1 {
                    n215 = call <vilib>:"Application Directory.vi"() -> ("Application Directory"=w227:path)
                    n216 = Build Path(base path=w227, name or relative path="data\\sys.ini" ("名称或相对路径")) -> (appended path=w229:path)
                    n217 = call <vilib>:"Open Config Data.vi"("configuration file path"=w229) -> ("error out"=w233:errorcluster, "refnum"=w230:T12)  [unwired: 8 in, 1 out]
                    n218 = vi-ref "断电保存全局.vi"() -> (w231:refnum<vi>)
                    n219 = call <userlib>:"Write Panel to INI__ogtk.vi"("error in (no error)"=w233, "VI ref"=w231, "refnum"=w230) -> ("error out"=w234:errorcluster, "refnum out"=w232:T12)  [unwired: 7 in]
                    n220 = call <vilib>:"Close Config Data.vi"("error in (no error)"=w234, "refnum"=w232) -> ("error out"=w239:errorcluster, "file path"=w240:path)  [unwired: 8 in]
                    n221 = Open/Create/Replace File(file path (use dialog)=w240, error in=w239) -> (refnum out=w236:refnum<file>, error out=w235:errorcluster)  [unwired: 4 in, 1 out]
                    n222 = Flush File(refnum=w236, error in=w235) -> (refnum out=w237:refnum<file>, error out=w238:errorcluster)
                    n223 = Close File(refnum=w237, error in=w238) -> ()  [unwired: 2 out]
                  }
                }
              }
            }
          }
          frame "数据发送协议" {
            n224 = Variant To Data(type=enum16{"2005-212协议", "2017-212协议"}."2017-212协议" ("数据"), Variant=w241) -> (data=w242:enum16{"2005-212协议", "2017-212协议"})  [unwired: 1 in, 1 out]
            n225 = global write "断电保存全局.vi" "数据发送协议"(w242) -> ()
            n226 = Two Button Dialog(message="2005对应旧版通信协议，2017对应最新版协议，对应协议因子编码会不同，\n更改可能导致数据不能被平台识别，确定更改数据发送协议吗？" ("消息")) -> (T button?=w245:bool)  [unwired: 2 in]
            n227 = case shown="真" w245 {
              tunnel: w244 -> [w249 _]
              frame False {
                n228 = Variant To Data(type=enum16{"2005-212协议", "2017-212协议"}."2017-212协议" ("数据"), Variant=w249) -> (data=w247:enum16{"2005-212协议", "2017-212协议"})  [unwired: 1 in, 1 out]
                n229 = global write "断电保存全局.vi" "数据发送协议"(w247) -> ()
              }
              frame True {
                n230 = call "配置文件断电保存(子VI).vi"() -> ()  [unwired: 12 in]
              }
            }
          }
          frame "数据组合发送" {
            n231 = Variant To Data(type=FALSE, Variant=w250) -> (data=w251:bool)  [unwired: 1 in, 1 out]
            n232 = global write "断电保存全局.vi" "数据组合发送"(w251) -> ()
            n233 = Two Button Dialog(message="勾选数据组合发送功能表示所有参数打包整点同时上传、则只能整点发送延时较高，\n不勾选则表示单参数分别上传、则实时性较好，确定更改数据组合发送功能吗？" ("消息")) -> (T button?=w254:bool)  [unwired: 2 in]
            n234 = case shown="真" w254 {
              tunnel: w253 -> [w257 _]
              frame False {
                n235 = Variant To Data(type=FALSE, Variant=w257) -> (data=w256:bool)  [unwired: 1 in, 1 out]
                n236 = global write "断电保存全局.vi" "数据组合发送"(w256) -> ()
              }
              frame True {
                n237 = flat-sequence {
                  frame #0 {
                  }
                  frame #1 {
                    n238 = call <vilib>:"Application Directory.vi"() -> ("Application Directory"=w259:path)
                    n239 = Build Path(base path=w259, name or relative path="data\\sys.ini" ("名称或相对路径")) -> (appended path=w261:path)
                    n240 = call <vilib>:"Open Config Data.vi"("configuration file path"=w261) -> ("error out"=w265:errorcluster, "refnum"=w262:T12)  [unwired: 8 in, 1 out]
                    n241 = vi-ref "断电保存全局.vi"() -> (w263:refnum<vi>)
                    n242 = call <userlib>:"Write Panel to INI__ogtk.vi"("error in (no error)"=w265, "VI ref"=w263, "refnum"=w262) -> ("error out"=w266:errorcluster, "refnum out"=w264:T12)  [unwired: 7 in]
                    n243 = call <vilib>:"Close Config Data.vi"("error in (no error)"=w266, "refnum"=w264) -> ("error out"=w271:errorcluster, "file path"=w272:path)  [unwired: 8 in]
                    n244 = Open/Create/Replace File(file path (use dialog)=w272, error in=w271) -> (refnum out=w268:refnum<file>, error out=w267:errorcluster)  [unwired: 4 in, 1 out]
                    n245 = Flush File(refnum=w268, error in=w267) -> (refnum out=w269:refnum<file>, error out=w270:errorcluster)
                    n246 = Close File(refnum=w269, error in=w270) -> ()  [unwired: 2 out]
                  }
                }
              }
            }
          }
          frame "自动更新" {
            n247 = Variant To Data(type=FALSE, Variant=w277) -> (data=w275:bool)  [unwired: 1 in, 1 out]
            n248 = global write "断电保存全局.vi" "自动更新"(w275) -> ()
            n249 = case shown="假" w275 {
              tunnel: ["关闭" "启用"] -> w274
              frame False {
              }
              frame True {
              }
            }
            n250 = Format Into String(format string="每周一0-6点间自动更新，确认%s？" ("消息"), w274) -> (resulting string=w273:string)  [unwired: 2 in, 1 out]
            n251 = Two Button Dialog(message=w273) -> (T button?=w280:bool)  [unwired: 2 in]
            n252 = case shown="真" w280 {
              tunnel: w279 -> [w284 _]
              frame False {
                n253 = Variant To Data(type=FALSE, Variant=w284) -> (data=w283:bool)  [unwired: 1 in, 1 out]
                n254 = global write "断电保存全局.vi" "自动更新"(w283) -> ()
              }
              frame True {
                n255 = flat-sequence {
                  frame #0 {
                  }
                  frame #1 {
                    n256 = call <vilib>:"Application Directory.vi"() -> ("Application Directory"=w286:path)
                    n257 = Build Path(base path=w286, name or relative path="data\\sys.ini" ("名称或相对路径")) -> (appended path=w288:path)
                    n258 = call <vilib>:"Open Config Data.vi"("configuration file path"=w288) -> ("error out"=w292:errorcluster, "refnum"=w289:T12)  [unwired: 8 in, 1 out]
                    n259 = vi-ref "断电保存全局.vi"() -> (w290:refnum<vi>)
                    n260 = call <userlib>:"Write Panel to INI__ogtk.vi"("error in (no error)"=w292, "VI ref"=w290, "refnum"=w289) -> ("error out"=w293:errorcluster, "refnum out"=w291:T12)  [unwired: 7 in]
                    n261 = call <vilib>:"Close Config Data.vi"("error in (no error)"=w293, "refnum"=w291) -> ("error out"=w298:errorcluster, "file path"=w299:path)  [unwired: 8 in]
                    n262 = Open/Create/Replace File(file path (use dialog)=w299, error in=w298) -> (refnum out=w295:refnum<file>, error out=w294:errorcluster)  [unwired: 4 in, 1 out]
                    n263 = Flush File(refnum=w295, error in=w294) -> (refnum out=w296:refnum<file>, error out=w297:errorcluster)
                    n264 = Close File(refnum=w296, error in=w297) -> ()  [unwired: 2 out]
                  }
                }
              }
            }
          }
          frame "2011发送" {
            n265 = Variant To Data(type=FALSE, Variant=w300) -> (data=w301:bool)  [unwired: 1 in, 1 out]
            n266 = global write "断电保存全局.vi" "2011发送"(w301) -> ()
            n267 = Two Button Dialog(message="2011表示实时数据上传，一般情况需要勾选，确定更改2011实时数据发送功能吗？" ("消息")) -> (T button?=w304:bool)  [unwired: 2 in]
            n268 = case shown="真" w304 {
              tunnel: w303 -> [w307 _]
              frame False {
                n269 = Variant To Data(type=FALSE, Variant=w307) -> (data=w306:bool)  [unwired: 1 in, 1 out]
                n270 = global write "断电保存全局.vi" "2011发送"(w306) -> ()
              }
              frame True {
                n271 = flat-sequence {
                  frame #0 {
                  }
                  frame #1 {
                    n272 = call <vilib>:"Application Directory.vi"() -> ("Application Directory"=w309:path)
                    n273 = Build Path(base path=w309, name or relative path="data\\sys.ini" ("名称或相对路径")) -> (appended path=w311:path)
                    n274 = call <vilib>:"Open Config Data.vi"("configuration file path"=w311) -> ("error out"=w315:errorcluster, "refnum"=w312:T12)  [unwired: 8 in, 1 out]
                    n275 = vi-ref "断电保存全局.vi"() -> (w313:refnum<vi>)
                    n276 = call <userlib>:"Write Panel to INI__ogtk.vi"("error in (no error)"=w315, "VI ref"=w313, "refnum"=w312) -> ("error out"=w316:errorcluster, "refnum out"=w314:T12)  [unwired: 7 in]
                    n277 = call <vilib>:"Close Config Data.vi"("error in (no error)"=w316, "refnum"=w314) -> ("error out"=w321:errorcluster, "file path"=w322:path)  [unwired: 8 in]
                    n278 = Open/Create/Replace File(file path (use dialog)=w322, error in=w321) -> (refnum out=w318:refnum<file>, error out=w317:errorcluster)  [unwired: 4 in, 1 out]
                    n279 = Flush File(refnum=w318, error in=w317) -> (refnum out=w319:refnum<file>, error out=w320:errorcluster)
                    n280 = Close File(refnum=w319, error in=w320) -> ()  [unwired: 2 out]
                  }
                }
              }
            }
          }
          frame "日志、参数发送" {
            n281 = Variant To Data(type=FALSE, Variant=w323) -> (data=w324:bool)  [unwired: 1 in, 1 out]
            n282 = global write "断电保存全局.vi" "日志、参数发送"(w324) -> ()
            n283 = Two Button Dialog(message="选择是否需要仪器日志、状态和告警信息上传，一般情况需要勾选，确定更改日志、参数发送功能吗？" ("消息")) -> (T button?=w327:bool)  [unwired: 2 in]
            n284 = case shown="假" w327 {
              tunnel: w326 -> [w330 _]
              frame False {
                n285 = Variant To Data(type=FALSE, Variant=w330) -> (data=w329:bool)  [unwired: 1 in, 1 out]
                n286 = global write "断电保存全局.vi" "日志、参数发送"(w329) -> ()
              }
              frame True {
                n287 = flat-sequence {
                  frame #0 {
                  }
                  frame #1 {
                    n288 = call <vilib>:"Application Directory.vi"() -> ("Application Directory"=w332:path)
                    n289 = Build Path(base path=w332, name or relative path="data\\sys.ini" ("名称或相对路径")) -> (appended path=w334:path)
                    n290 = call <vilib>:"Open Config Data.vi"("configuration file path"=w334) -> ("error out"=w338:errorcluster, "refnum"=w335:T12)  [unwired: 8 in, 1 out]
                    n291 = vi-ref "断电保存全局.vi"() -> (w336:refnum<vi>)
                    n292 = call <userlib>:"Write Panel to INI__ogtk.vi"("error in (no error)"=w338, "VI ref"=w336, "refnum"=w335) -> ("error out"=w339:errorcluster, "refnum out"=w337:T12)  [unwired: 7 in]
                    n293 = call <vilib>:"Close Config Data.vi"("error in (no error)"=w339, "refnum"=w337) -> ("error out"=w344:errorcluster, "file path"=w345:path)  [unwired: 8 in]
                    n294 = Open/Create/Replace File(file path (use dialog)=w345, error in=w344) -> (refnum out=w341:refnum<file>, error out=w340:errorcluster)  [unwired: 4 in, 1 out]
                    n295 = Flush File(refnum=w341, error in=w340) -> (refnum out=w342:refnum<file>, error out=w343:errorcluster)
                    n296 = Close File(refnum=w342, error in=w343) -> ()  [unwired: 2 out]
                  }
                }
              }
            }
          }
          frame "判断数据反馈" {
            n297 = Two Button Dialog(message="判断数据反馈是针对平台能有反馈的情况，\n1.严格判断反馈-收不到反馈一直重发\n2.非严格判断-重发5次后跳过该数据\n3.不判断反馈针对平台没有反馈的情况\n确定更改判断数据反馈功能吗？" ("消息")) -> (T button?=w348:bool)  [unwired: 2 in]
            n298 = case shown="假" w348 {
              tunnel: w347 -> [_ _]
              tunnel: w346 -> [w351 w353]
              frame False {
                n299 = Variant To Data(type=enum16{"非严格判断", "严格判断", "不判断"}."非严格判断" ("判断数据反馈"), Variant=w351) -> (data=w350:enum16{"非严格判断", "严格判断", "不判断"})  [unwired: 1 in, 1 out]
                n300 = local write "判断数据反馈"(w350) -> ()
              }
              frame True {
                n301 = flat-sequence {
                  tunnel: w353 -> [w354]
                  frame #0 {
                    n302 = Variant To Data(type=enum16{"非严格判断", "严格判断", "不判断"}."非严格判断" ("判断数据反馈"), Variant=w354) -> (data=w356:enum16{"非严格判断", "严格判断", "不判断"})  [unwired: 1 in, 1 out]
                    n303 = global write "断电保存全局.vi" "判断数据反馈"(w356) -> ()
                  }
                  frame #1 {
                    n304 = call <vilib>:"Application Directory.vi"() -> ("Application Directory"=w357:path)
                    n305 = Build Path(base path=w357, name or relative path="data\\sys.ini" ("名称或相对路径")) -> (appended path=w359:path)
                    n306 = call <vilib>:"Open Config Data.vi"("configuration file path"=w359) -> ("error out"=w363:errorcluster, "refnum"=w360:T12)  [unwired: 8 in, 1 out]
                    n307 = vi-ref "断电保存全局.vi"() -> (w361:refnum<vi>)
                    n308 = call <userlib>:"Write Panel to INI__ogtk.vi"("error in (no error)"=w363, "VI ref"=w361, "refnum"=w360) -> ("error out"=w364:errorcluster, "refnum out"=w362:T12)  [unwired: 7 in]
                    n309 = call <vilib>:"Close Config Data.vi"("error in (no error)"=w364, "refnum"=w362) -> ("error out"=w369:errorcluster, "file path"=w370:path)  [unwired: 8 in]
                    n310 = Open/Create/Replace File(file path (use dialog)=w370, error in=w369) -> (refnum out=w366:refnum<file>, error out=w365:errorcluster)  [unwired: 4 in, 1 out]
                    n311 = Flush File(refnum=w366, error in=w365) -> (refnum out=w367:refnum<file>, error out=w368:errorcluster)
                    n312 = Close File(refnum=w367, error in=w368) -> ()  [unwired: 2 out]
                  }
                }
              }
            }
          }
        }
      }
      event "确定": Value Change {
        n313 = event-data() -> ()  [unwired: 1 in, 6 out]
        n314 = call "通信状态入队列.vi"("枚举"=enum16{"打开连接", "发送数据", "读取数据", "数据处理", "关闭连接"}."关闭连接") -> ()  [unwired: 10 in, 1 out]
      }
      event "配置表": Value Change {
        n315 = event-data() -> ()  [unwired: 1 in, 6 out]
        n316 = call "参数配置表.vi"() -> ()  [unwired: 12 in]
      }
      event "参数配置": Value Change {
        n317 = event-data() -> ()  [unwired: 1 in, 6 out]
        n318 = property on="窗格" class="Pane"("Origin"=T7 {"Horizontal"=0, "Vertical"=1000} ("原点")) -> ()  [unwired: 2 in, 2 out]
        n319 = call <vilib>:"Application Directory.vi"() -> ("Application Directory"=w378:path)
        n320 = call "查询启动项.vi"("启动文件路径"=w378) -> ("error out"=w373:errorcluster, "包含启动项"=w377:bool)  [unwired: 9 in]
        n321 = local write "开机启动"(w377) -> ()
        n322 = local read "MN"() -> (w376:string)
        n323 = local read "PW"() -> (w375:string)
        n324 = Bundle("MN"=w376, "PW"=w375) -> (w374:cluster{"MN":string, "PW":string})  [unwired: 1 in]
        n325 = call "查询MN号.vi"("error in (no error)"=w373, "簇"=w374) -> ("包含启动项"=w372:bool)  [unwired: 8 in, 1 out]
        n326 = local write "共享MN"(w372) -> ()
      }
      event "返回": Value Change {
        n327 = event-data() -> ()  [unwired: 1 in, 6 out]
        n328 = property on="窗格" class="Pane"("Origin"=T7 {"Horizontal"=0, "Vertical"=0} ("原点")) -> ()  [unwired: 2 in, 2 out]
      }
      event "数据补传": Value Change {
        n329 = event-data() -> ()  [unwired: 1 in, 6 out]
        n330 = global read "全局1.vi" "数据发送起始时间"() -> (w383:timestamp)
        n331 = call "数据补传对话框.vi"("起始时间"=w383) -> ("参数数值out"=w382:T13, "结束时间输出"=w384:timestamp, "起始时间输出"=w385:timestamp, "输出"=w386:bool, "只补小时数据输出"=w381:bool)  [unwired: 6 in]
        n332 = case shown="真" w386 {
          tunnel: w385 -> [_ w395]
          tunnel: w384 -> [_ w396]
          tunnel: w382 -> [_ w392]
          tunnel: w381 -> [_ w394]
          frame False {
          }
          frame True {
            w393 = TRUE ("数据重发")
            n333 = global read "全局 水样时间.vi" "水样数据索引"() -> (w391:T14)
            n334 = global write "全局1.vi" "数据发送起始时间"(w395) -> ()
            n335 = global write "断电保存全局.vi" "数据重发结束时间"(w396) -> ()
            n336 = Cluster To Array(cluster=w392) -> (array=w390:bool[])
            n337 = global write "断电保存全局.vi" "数据重发"(w393) -> ()
            n338 = Cluster To Array(cluster=w391) -> (array=w389:string[])
            n339 = Format Date/Time String(time format string (%c)="%Y/%m/%d %H:%M:%S" ("时间格式字符串(%c)"), seconds (now)=w395) -> (date/time string=w388:string)  [unwired: 1 in]
            n340 = for {
              tunnel: w390 -> [w402] mode=indexing
              tunnel: w389 -> [w400] mode=indexing
              tunnel: w388 -> [w401]
              tunnel: [w399] -> w387 mode=indexing
              n341 = Select(t=w401, s=w402, f=w400) -> (s? t:f=w399:string)
            }
            n342 = case shown="假" w394 {
              tunnel: w388 -> [w410 _]
              tunnel: w393 -> [w403 _]
              frame False {
                n343 = global read "断电保存全局.vi" "数据组合发送"() -> (w411:bool)
                n344 = global write "全局 水样时间.vi" "剖面数据时间"(w410) -> ()
                n345 = global write "断电保存全局.vi" "数据重发时间戳"(w410) -> ()
                n346 = Initialize Array(w410, 8 ("维数大小")) -> (w406:string[])
                n347 = Initialize Array(w410, 15 ("维数大小")) -> (w407:string[])
                n348 = global write "全局 水样时间.vi" "剖面多参数数据时间"(w410) -> ()
                n349 = case shown="假" w411 {
                  tunnel: w410 -> [w412 _]
                  frame False {
                    n350 = global write "全局 时间2.vi" "标样核查索引起始时间"(w412) -> ()
                    n351 = global write "全局 时间2.vi" "加标回收索引起始时间"(w412) -> ()
                    n352 = global write "全局 时间2.vi" "跨度核查索引起始时间"(w412) -> ()
                    n353 = global write "全局 时间2.vi" "3092日志索引起始时间"(w412) -> ()
                    n354 = global write "全局 时间2.vi" "零点核查索引起始时间"(w412) -> ()
                    n355 = Initialize Array(w412, 10 ("维数大小")) -> (w424:string[])
                    n356 = Initialize Array(w412, 7 ("维数大小")) -> (w416:string[])
                    n357 = Initialize Array(w412, 8 ("维数大小")) -> (w415:string[])
                    n358 = Initialize Array(w412, 18 ("维数大小")) -> (w419:string[])
                    n359 = Array To Cluster(array=w415) -> (cluster=w414:T15)
                    n360 = Array To Cluster(array=w424) -> (cluster=w423:T16)
                    n361 = Array To Cluster(array=w416) -> (cluster=w417:T17)
                    n362 = global write "全局 时间2.vi" "跨度核查索引"(w423) -> ()
                    n363 = global write "全局 时间2.vi" "零点核查索引"(w423) -> ()
                    n364 = global write "全局 时间2.vi" "平行样索引"(w417) -> ()
                    n365 = global write "全局 时间2.vi" "加标回收索引"(w417) -> ()
                    n366 = global write "全局 时间2.vi" "仪器日志索引"(w414) -> ()
                    n367 = Array To Cluster(array=w419) -> (cluster=w420:T18)
                    n368 = global write "全局 时间2.vi" "标样核查索引"(w420) -> ()
                    n369 = global write "全局 时间2.vi" "集成干预索引"(w420) -> ()
                  }
                  frame True {
                  }
                }
                n370 = Array To Cluster(array=w406) -> (cluster=w405:T15)
                n371 = global write "全局 时间2.vi" "仪器日志索引"(w405) -> ()
                n372 = Array To Cluster(array=w407) -> (cluster=w408:T19)
                n373 = global write "断电保存全局.vi" "日志信息重发"(w403) -> ()
                n374 = global write "断电保存全局.vi" "剖面数据重发"(w403) -> ()
                n375 = global write "全局 时间2.vi" "仪器参数索引"(w408) -> ()
              }
              frame True {
                n376 = global write "断电保存全局.vi" "2011发送"(FALSE ("2011发送")) -> ()
              }
            }
            n377 = Array To Cluster(array=w387) -> (cluster=w397:T20)
            n378 = global write "全局 水样时间.vi" "水样数据索引"(w397) -> ()
          }
        }
      }
      event "开机启动": Value Change {
        n379 = event-data() -> ("CtlRef"=w427:refnum<vi>, "OldVal"=w426:bool, "NewVal"=w428:bool)  [unwired: 1 in, 3 out]
        n380 = case shown="假" w428 {
          tunnel: w427 -> [w430 w443]
          tunnel: w426 -> [w429 w442]
          frame False {
            n381 = Two Button Dialog(message="是否删除开机启动？" ("消息"), 1:"否" ("F按钮名称（“取消”）"), 2:"是" ("T按钮名称（“确定”）")) -> (T button?=w431:bool)
            n382 = case shown="真" w431 {
              tunnel: w430 -> [w436 _]
              tunnel: w429 -> [w435 _]
              frame False {
                n383 = property class="Bool (严格)"(reference=w436, "Value"=w435) -> ()  [unwired: 1 in, 2 out]
              }
              frame True {
                n384 = call <vilib>:"Application Directory.vi"() -> ("Application Directory"=w438:path)
                n385 = call "删除启动项.vi"("启动文件路径"=w438) -> ("删除标记"=w437:bool)  [unwired: 9 in, 1 out]
                n386 = case shown="真" w437 {
                  tunnel: ["删除开机启动失败" ("T按钮名称（“确定”）") "删除开机启动成功" ("T按钮名称（“确定”）")] -> w439
                  frame False {
                  }
                  frame True {
                  }
                }
                n387 = One Button Dialog(message=w439) -> ()  [unwired: 1 in, 1 out]
              }
            }
          }
          frame True {
            n388 = Two Button Dialog(message="是否添加开机启动？" ("消息"), 1:"否" ("F按钮名称（“取消”）"), 2:"是" ("T按钮名称（“确定”）")) -> (T button?=w444:bool)
            n389 = case shown="真" w444 {
              tunnel: w443 -> [w449 _]
              tunnel: w442 -> [w448 _]
              frame False {
                n390 = property class="Bool (严格)"(reference=w449, "Value"=w448) -> ()  [unwired: 1 in, 2 out]
              }
              frame True {
                n391 = call <vilib>:"Application Directory.vi"() -> ("Application Directory"=w452:path)
                n392 = call "添加启动项.vi"("启动文件路径"=w452) -> ("添加成功标记"=w451:bool)  [unwired: 9 in, 1 out]
                n393 = case shown="真" w451 {
                  tunnel: ["添加开机启动失败" ("T按钮名称（“确定”）") "添加开机启动成功" ("T按钮名称（“确定”）")] -> w450
                  frame False {
                  }
                  frame True {
                  }
                }
                n394 = One Button Dialog(message=w450) -> ()  [unwired: 1 in, 1 out]
              }
            }
          }
        }
      }
      event "共享MN": Value Change {
        n395 = event-data() -> ("CtlRef"=w456:refnum<vi>, "OldVal"=w455:bool, "NewVal"=w457:bool)  [unwired: 1 in, 3 out]
        n396 = case shown="真" w457 {
          tunnel: w456 -> [w459 w474]
          tunnel: w455 -> [w458 w473]
          frame False {
            n397 = Two Button Dialog(message="是否取消该MN号共享？" ("消息"), 1:"否" ("F按钮名称（“取消”）"), 2:"是" ("T按钮名称（“确定”）")) -> (T button?=w460:bool)
            n398 = case shown="真" w460 {
              tunnel: w459 -> [w465 _]
              tunnel: w458 -> [w464 _]
              frame False {
                n399 = property class="Bool (严格)"(reference=w465, "Value"=w464) -> ()  [unwired: 1 in, 2 out]
              }
              frame True {
                n400 = local read "MN"() -> (w469:string)
                n401 = local read "PW"() -> (w468:string)
                n402 = Bundle("MN"=w469, "PW"=w468) -> (w467:cluster{"MN":string, "PW":string})  [unwired: 1 in]
                n403 = call "删除MN号.vi"("簇"=w467) -> ("删除标记"=w466:bool)  [unwired: 9 in, 1 out]
                n404 = case shown="真" w466 {
                  tunnel: ["取消该MN号共享失败" ("T按钮名称（“确定”）") "取消该MN号共享成功" ("T按钮名称（“确定”）")] -> w470
                  frame False {
                  }
                  frame True {
                  }
                }
                n405 = One Button Dialog(message=w470) -> ()  [unwired: 1 in, 1 out]
              }
            }
          }
          frame True {
            n406 = Two Button Dialog(message="是否添加该MN号共享？" ("消息"), 1:"否" ("F按钮名称（“取消”）"), 2:"是" ("T按钮名称（“确定”）")) -> (T button?=w475:bool)
            n407 = case shown="真" w475 {
              tunnel: w474 -> [w480 _]
              tunnel: w473 -> [w479 _]
              frame False {
                n408 = property class="Bool (严格)"(reference=w480, "Value"=w479) -> ()  [unwired: 1 in, 2 out]
              }
              frame True {
                n409 = local read "MN"() -> (w484:string)
                n410 = local read "PW"() -> (w483:string)
                n411 = Bundle("MN"=w484, "PW"=w483) -> (w482:cluster{"MN":string, "PW":string})  [unwired: 1 in]
                n412 = call "添加MN号.vi"("簇"=w482) -> ("添加成功标记"=w481:bool)  [unwired: 9 in, 1 out]
                n413 = case shown="假" w481 {
                  tunnel: ["添加该MN号共享失败" ("T按钮名称（“确定”）") "添加该MN号共享成功" ("T按钮名称（“确定”）")] -> w485
                  frame False {
                  }
                  frame True {
                  }
                }
                n414 = One Button Dialog(message=w485) -> ()  [unwired: 1 in, 1 out]
              }
            }
          }
        }
      }
      event "更新": Value Change {
        n415 = event-data() -> ()  [unwired: 1 in, 6 out]
        n416 = call "自定义双按钮对话框.vi"("消息"="选择是否从服务器获取最新版本信息？") -> ("正式版/测试版输出"=w488:bool, "输出"=w489:bool)  [unwired: 9 in]
        n417 = case shown="真" w489 {
          tunnel: w488 -> [_ w493]
          frame False {
          }
          frame True {
            w500 = T21 2 items=["两端", "字符串首端", "字符串末端"] ("location (both)")
            w498 = "/" ("分隔符(Tab)")
            # "获取最新版本"
            n418 = local read "updateconfiguration"() -> (w504:T1)
            n419 = Unbundle By Name(w504) -> ("远程路径"=w492:string)
            n420 = Spreadsheet String To Array(delimiter (Tab)="\\" ("分隔符(Tab)"), format string="" ("格式字符串"), spreadsheet string=w492, array type (2D Dbl)=string[] []) -> (array=w495:string[])
            n421 = case shown="真" w493 {
              tunnel: w495 -> [w505 w507]
              tunnel: [w505 w506] -> w494
              frame False {
                # "正式版"
              }
              frame True {
                # "测试版"
                n422 = Array Size(array=w507) -> (size(s)=w508:i32)
                n423 = Subtract(x=w508, y=2) -> (x-y=w510:i32)
                n424 = Index Array(array=w507, index=w510) -> (element=w511:string)
                n425 = Concatenate Strings(w511, "beta" ("字符串")) -> (w513:string)
                n426 = Replace Array Subset(array=w507, new element=w513, index=w510) -> (w506:string[])
              }
            }
            n427 = Array To Spreadsheet String(delimiter (Tab)=w498, array=w494, 3:"%s" ("格式字符串")) -> (spreadsheet string=w497:string)
            n428 = Concatenate Strings(w498, w497) -> (w496:string)
            n429 = call <vilib>:"Trim Whitespace.vi"("string"=w496, "location (both)"=w500) -> ("trimmed string"=w491:string)
            n430 = call "Updateinter.vi"("更新包远端地址"=w491, "测试版？"=w493) -> ()  [unwired: 10 in]
          }
        }
      }
      event "IP", "PORT": Mouse Down {
        n431 = event-data() -> ("CtlRef"=w522:refnum<vi>)  [unwired: 1 in, 7 out]
        n432 = property class="Str"(reference=w522) -> (reference out=w520:refnum<vi>, "Value"=w521:string)  [unwired: 1 in, 1 out]
        n433 = call "IP键盘.vi"("OldNumber"=w521) -> ("NewNumber"=w517:string)
        n434 = String Length(string=w517) -> (length=w519:i32)
        n435 = Less Or Equal?(x=w519, y=50) -> (x <= y?=w516:bool)
        n436 = case shown="假" w516 {
          tunnel: w520 -> [w523 w527]
          tunnel: w517 -> [_ w526]
          tunnel: [w523 w527] -> w515
          tunnel: ["127.0.0.1" w526] -> w514
          frame False {
            n437 = One Button Dialog(message="超过ipv4最大长度限制,请重新输入!" ("消息")) -> ()  [unwired: 1 in, 1 out]
          }
          frame True {
          }
        }
        n438 = property class="Str"(reference=w515, "Val(Sgnl)"=w514) -> ()  [unwired: 1 in, 2 out]
      }
    }
  }
  n439 = while {
    shift-right: [w532] -> _
    shift-left: "数  据  采  集  传  输  系  统" ("标题显示") -> [w533]
    stop <- FALSE stop-if-true
    n440 = global read "断电保存全局.vi" "数据重发"() -> (w530:bool)
    n441 = global read "断电保存全局.vi" "日志信息重发"() -> (w529:bool)
    n442 = global read "断电保存全局.vi" "剖面数据重发"() -> (w528:bool)
    n443 = call "字符串移位显示.vi"("字符框大小"=72, "字符串输入"=w533) -> ("移位后字符串"=w532:string)  [unwired: 8 in, 1 out]
    "标题显示" <- w532
    n444 = Wait (ms)(milliseconds to wait=u32 1000 ("等待时间（毫秒）")) -> ()  [unwired: 1 out]
    n445 = property on="数据补发" class="Bool (严格)"("Visible"=w530, "Value"=w530) -> ()  [unwired: 2 in, 2 out]
    n446 = property on="日志信息补发" class="Bool (严格)"("Visible"=w529, "Value"=w529) -> ()  [unwired: 2 in, 2 out]
    n447 = property on="剖面数据补发" class="Bool (严格)"("Visible"=w528, "Value"=w528) -> ()  [unwired: 2 in, 2 out]
  }
